vi "Clear Methods Registration.vi"(8 "error in (no error)":errorcluster, 11 "Server class in":refnum<vi>) -> (0 "error out":errorcluster, 3 "Server class out":refnum<vi>)   [LabVIEW 2019, in "gRPC Scripting Tools.lvlib"]
uses:
  gRPC Scripting Tools.lvlib
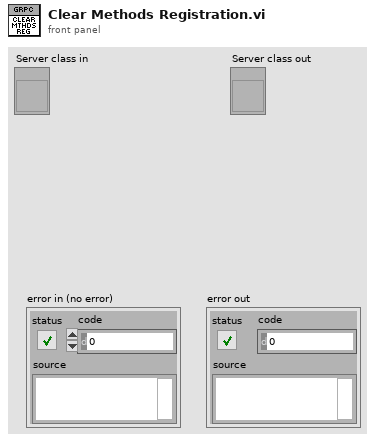
[diagram p1: front panel]
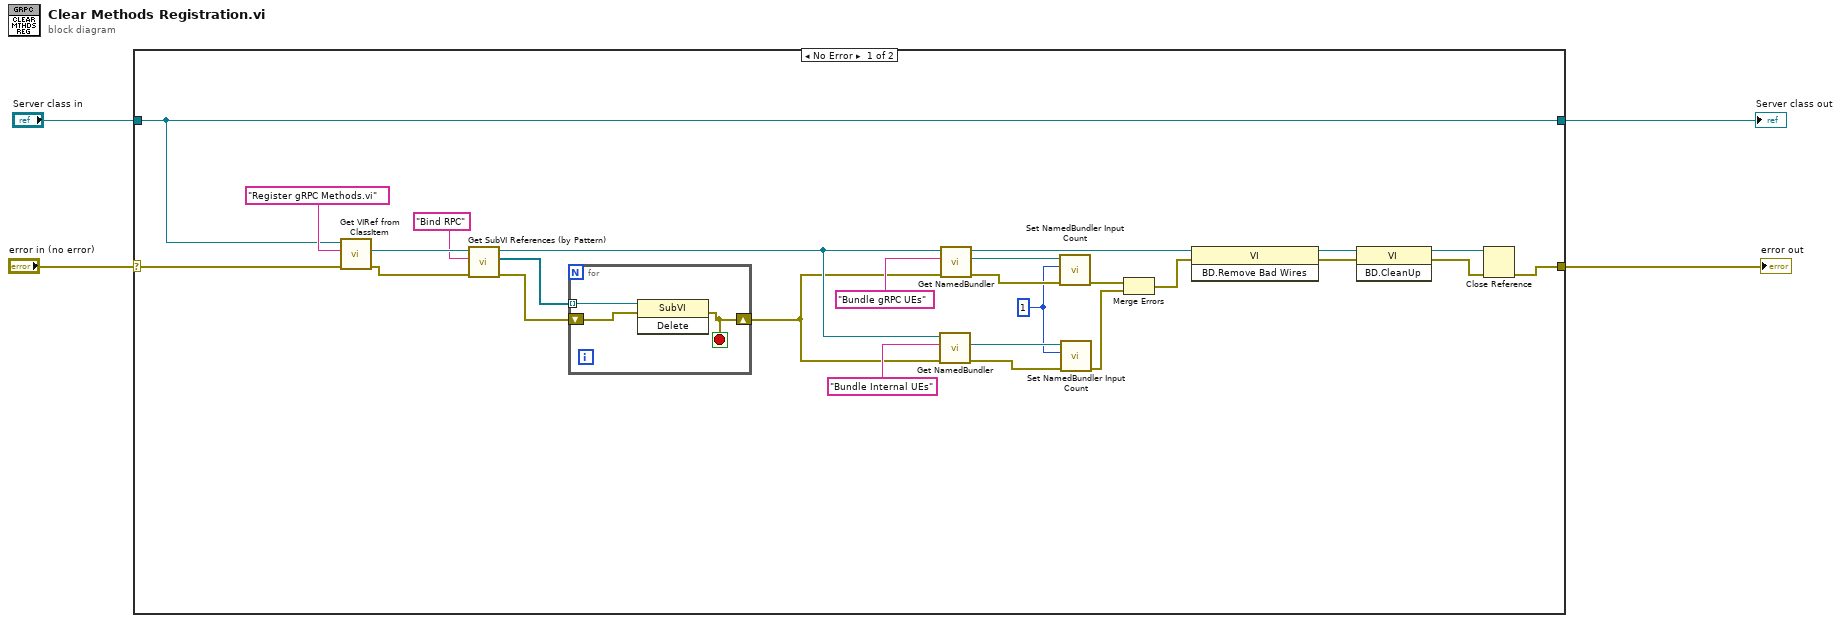
[diagram p0: block diagram]
diagram:
  n1 = case shown="No Error" "error in (no error)" {
    selector: "error in (no error)" -> [w29 w34]
    tunnel: [w18 w34] -> w4
    tunnel: "Server class in" -> [w28 w35]
    tunnel: [w28 w35] -> w1
    frame No Error {
      w8 = 1 ("Numeric")
      n2 = call "Get VIRef from ClassItem.vi"("error in (no error)"=w29, "Item Name"="Register gRPC Methods.vi", "LVClassLibrary in"=w28) -> ("error out"=w27:errorcluster, "VIref out"=w26:refnum<vi>)  [unwired: 5 in, 2 out]
      n3 = call "Get SubVI References (by Pattern).vi"("error in (no error)"=w27, "SubVI Name Pattern"="Bind RPC" ("regular expression"), "VI ref in"=w26) -> ("error out"=w24:errorcluster, "SubVI refs"=w23:refnum<vi>[], "VI ref out"=w11:refnum<vi>)  [unwired: 6 in]
      n4 = for {
        tunnel: w23 -> [w33] mode=indexing
        shift-right: [w31] -> w9
        shift-left: w24 -> [w32]
        stop <- w31 stop-if-true
        n5 = invoke class="SubVI" method="Delete"(reference=w33, error in=w32) -> (error out=w31:errorcluster)  [unwired: 1 in, 2 out]
      }
      n6 = call "Get NamedBundler.vi"("error in (no error)"=w9, "Label"="Bundle Internal UEs" ("name/order"), "Owner VI in"=w11) -> ("error out"=w13:errorcluster, "NamedBundler ref out"=w14:refnum<vi>)  [unwired: 5 in, 2 out]
      n7 = call "Get NamedBundler.vi"("error in (no error)"=w9, "Label"="Bundle gRPC UEs" ("name/order"), "Owner VI in"=w11) -> ("error out"=w15:errorcluster, "NamedBundler ref out"=w17:refnum<vi>, "Owner VI out"=w12:refnum<vi>)  [unwired: 5 in, 1 out]
      n8 = call "Set NamedBundler Input Count.vi"("error in (no error)"=w15, "Numeric"=w8, "NamedBundler in"=w17) -> ("error out"=w7:errorcluster)  [unwired: 7 in, 1 out]
      n9 = call "Set NamedBundler Input Count.vi"("error in (no error)"=w13, "Numeric"=w8, "NamedBundler in"=w14) -> ("error out"=w6:errorcluster)  [unwired: 7 in, 1 out]
      n10 = Merge Errors(w7, w6) -> (w5:errorcluster)
      n11 = invoke class="VI" method="BD.Remove Bad Wires"(reference=w12, error in=w5) -> (reference out=w22:refnum<vi>, error out=w21:errorcluster)  [unwired: 1 in, 1 out]
      n12 = invoke class="VI" method="BD.CleanUp"(reference=w22, error in=w21) -> (reference out=w19:refnum<vi>, error out=w20:errorcluster)  [unwired: 1 in, 1 out]
      n13 = Close Reference(reference=w19, error in (no error)=w20) -> (error out=w18:errorcluster)
    }
    frame Error {
    }
  }
  "error out" <- w4
  "Server class out" <- w1
